vi "Menu.vi"() -> ()   [LabVIEW 2017]
panel:
  in  "OK Button":bool
  in  "Enum":enum16{"OFET", "OLED", "OLET", "OPV"}(ring)
  # "Bienvenido a la estación de prueba para \ndispositivos orgánicos"
  # "¿Qué dispositivo deseas analizar?"
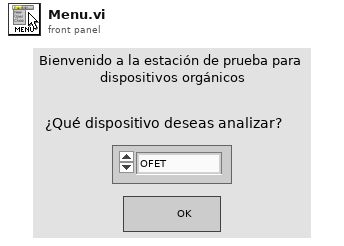
[diagram p1: front panel]
types:
  T1 = enum32{"Invalid", "Standard", "Closed", "Hidden", "Minimized", "Maximized"}
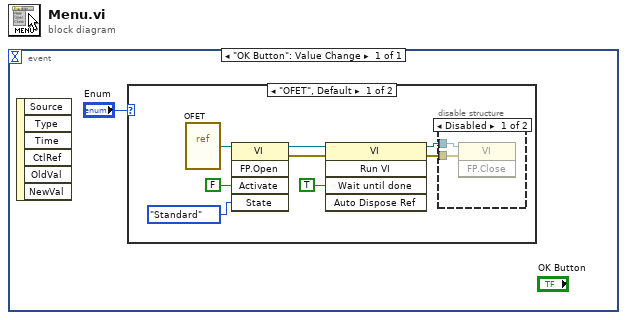
[diagram p0: block diagram]
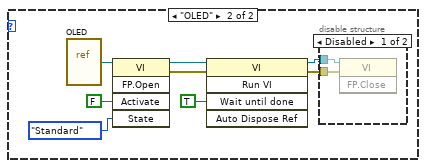
[diagram p3: hidden frame]
diagram:
  n1 = event shown="[0] \"OK Button\": Value Change" {
    selector: _ -> [_]
    dyn-events: _ -> [_]
    timeout: _ -> [_]
    event "OK Button": Value Change {
      n2 = event-data() -> ()  [unwired: 1 in, 6 out]
      n3 = case shown="\"OFET\", Default" "Enum" {
        frame "OFET", Default {
          n4 = vi-ref "OFET.vi"() -> (w2:refnum<vi>)
          n5 = invoke class="VI" method="FP.Open"(reference=w2, "Activate"=FALSE ("Activate?"), "State"=T1."Standard") -> (reference out=w8:refnum<vi>, error out=w7:errorcluster)  [unwired: 2 in, 3 out]
          n6 = invoke class="VI" method="Run VI"(reference=w8, error in=w7, "Wait until done"=TRUE) -> (reference out=w4:refnum<vi>, error out=w3:errorcluster)  [unwired: 2 in, 3 out]
          n7 = disable-structure shown="Disabled" {
            disable-tunnel: w4 -> [w11 _]
            disable-tunnel: w3 -> [w10 _]
            frame Disabled {
              n8 = invoke class="VI" method="FP.Close"(reference=w11, error in=w10) -> ()  [unwired: 1 in, 3 out]
            }
            frame Enabled {
            }
          }
        }
        frame "OLED" {
          n9 = vi-ref "OLED.vi"() -> (w19:refnum<vi>)
          n10 = invoke class="VI" method="FP.Open"(reference=w19, "Activate"=FALSE ("Activate?"), "State"=T1."Standard") -> (reference out=w17:refnum<vi>, error out=w16:errorcluster)  [unwired: 2 in, 3 out]
          n11 = invoke class="VI" method="Run VI"(reference=w17, error in=w16, "Wait until done"=TRUE) -> (reference out=w13:refnum<vi>, error out=w12:errorcluster)  [unwired: 2 in, 3 out]
          n12 = disable-structure shown="Disabled" {
            disable-tunnel: w13 -> [w21 _]
            disable-tunnel: w12 -> [w20 _]
            frame Disabled {
              n13 = invoke class="VI" method="FP.Close"(reference=w21, error in=w20) -> ()  [unwired: 1 in, 3 out]
            }
            frame Enabled {
            }
          }
        }
      }
    }
  }
